vi "MISC Wait on Queue From Multiple.vi"(0 "Queue A":refnum<queue>, 5 "Queue B":refnum<queue>, 7 "timeout in ms (-1)":i32=-1, 11 "error in (no error)":errorcluster) -> (4 "Queue Element":string, 6 "Queue A?":bool, 8 "Queue B?":bool, 10 "Timed Out":bool, 15 "error Out":errorcluster)   [LabVIEW 2011]
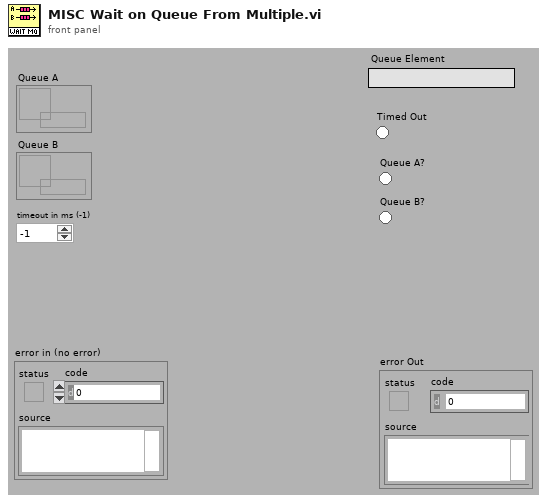
[diagram p1: front panel]
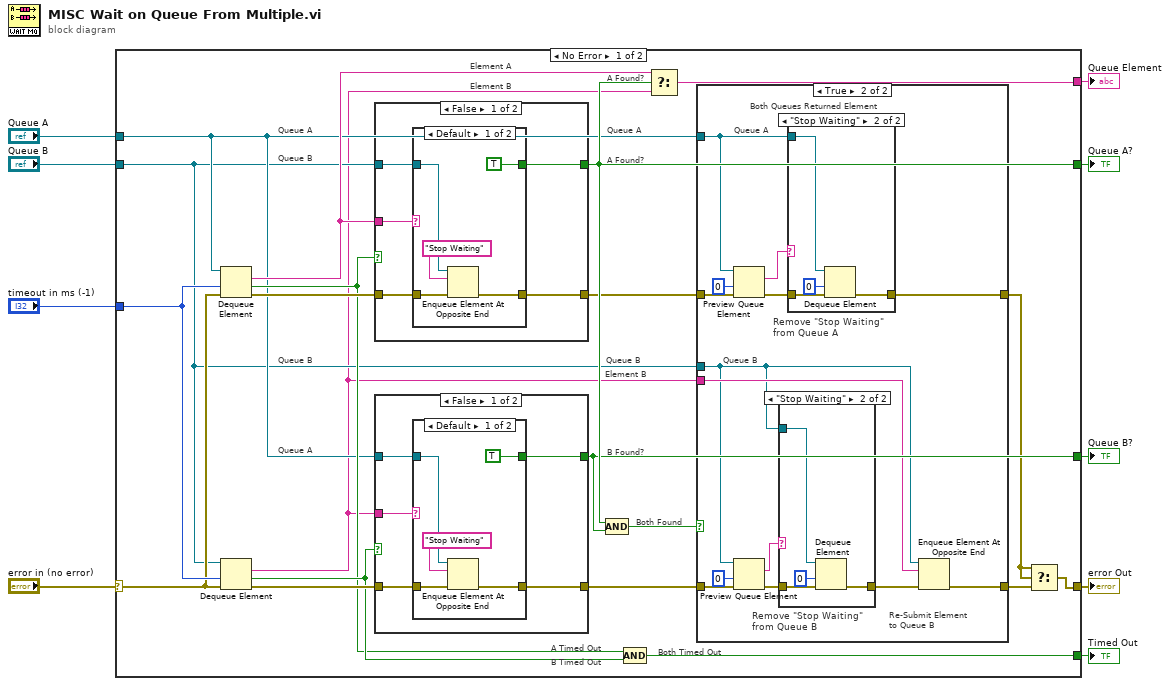
[diagram p0: block diagram]
diagram:
  n1 = case shown="No Error" "error in (no error)" {
    selector: "error in (no error)" -> [w28 w79]
    tunnel: "Queue B" -> [w14 _]
    tunnel: "Queue A" -> [w15 _]
    tunnel: "timeout in ms (-1)" -> [w29 _]
    tunnel: [w10 w79] -> w6
    tunnel: [w22 _] -> w4
    tunnel: [w21 _] -> w3
    tunnel: [w25 _] -> w2
    tunnel: [w23 _] -> w1
    frame No Error {
      # "Both Timed Out"
      # "Both Found"
      # "B Found?"
      # "Queue B"
      # "Element B"
      # "Queue A"
      # "A Found?"
      # "A Found?"
      # "Element B"
      # "Element A"
      # "B Timed Out"
      # "A Timed Out"
      # "Queue A"
      # "Queue B"
      # "Queue B"
      # "Queue A"
      n2 = Dequeue Element(queue=w15, timeout in ms (-1)=w29, error in (no error)=w28) -> (element=w24:string, timed out?=w18:bool, error out=w27:errorcluster)  [unwired: 1 out]
      n3 = Dequeue Element(queue=w14, timeout in ms (-1)=w29, error in (no error)=w28) -> (element=w13:string, timed out?=w19:bool, error out=w26:errorcluster)  [unwired: 1 out]
      n4 = case shown="False" w18 {
        tunnel: w14 -> [w71 _]
        tunnel: w27 -> [w70 w78]
        tunnel: w24 -> [w69 _]
        tunnel: [w68 w78] -> w17
        tunnel: [w67 _] -> w22
        frame False {
          n5 = case shown="Default" w69 {
            tunnel: w70 -> [w76 w77]
            tunnel: w71 -> [w75 _]
            tunnel: [w73 w77] -> w68
            tunnel: [TRUE _] -> w67
            frame Default {
              n6 = Enqueue Element At Opposite End(queue=w75, element="Stop Waiting", error in (no error)=w76) -> (error out=w73:errorcluster)  [unwired: 3 out]
            }
            frame "Stop Waiting" {
            }
          }
        }
        frame True {
        }
      }
      n7 = case shown="False" w19 {
        tunnel: w15 -> [w59 _]
        tunnel: w26 -> [w58 w66]
        tunnel: w13 -> [w57 _]
        tunnel: [w56 w66] -> w16
        tunnel: [w55 _] -> w21
        frame False {
          n8 = case shown="Default" w57 {
            tunnel: w58 -> [w64 w65]
            tunnel: w59 -> [w63 _]
            tunnel: [w61 w65] -> w56
            tunnel: [TRUE _] -> w55
            frame Default {
              n9 = Enqueue Element At Opposite End(queue=w63, element="Stop Waiting", error in (no error)=w64) -> (error out=w61:errorcluster)  [unwired: 3 out]
            }
            frame "Stop Waiting" {
            }
          }
        }
        frame True {
        }
      }
      n10 = Compound Arithmetic op=AND(w22, w21) -> (w20:bool)
      n11 = Compound Arithmetic op=AND(w18, w19) -> (w25:bool)
      n12 = Select(t=w24, s=w22, f=w13) -> (s? t:f=w23:string)
      n13 = case shown="True" w20 {
        tunnel: w16 -> [w31 w42]
        tunnel: [w31 w44] -> w11
        tunnel: w17 -> [w30 w43]
        tunnel: w15 -> [_ w38]
        tunnel: w14 -> [_ w33]
        tunnel: w13 -> [_ w41]
        tunnel: [w30 w37] -> w12
        frame False {
          # "0 or 1 Queues returned an Element"
        }
        frame True {
          # "Re-Submit Element to Queue B"
          # "Remove \"Stop Waiting\" from Queue A"
          # "Remove \"Stop Waiting\" from Queue B"
          # "Both Queues Returned Element"
          # "Queue B"
          # "Queue A"
          n14 = Preview Queue Element(queue=w38, timeout in ms (-1)=0, error in (no error)=w43) -> (element=w40:string, error out=w39:errorcluster)  [unwired: 2 out]
          n15 = Preview Queue Element(queue=w33, timeout in ms (-1)=0, error in (no error)=w42) -> (element=w32:string, error out=w34:errorcluster)  [unwired: 2 out]
          n16 = case shown="\"Stop Waiting\"" w32 {
            tunnel: w34 -> [w45 w49]
            tunnel: w33 -> [_ w48]
            tunnel: [w45 w46] -> _
            frame Default {
            }
            frame "Stop Waiting" {
              n17 = Dequeue Element(queue=w48, timeout in ms (-1)=0, error in (no error)=w49) -> (error out=w46:errorcluster)  [unwired: 3 out]
            }
          }
          n18 = case shown="\"Stop Waiting\"" w40 {
            tunnel: w39 -> [w50 w54]
            tunnel: w38 -> [_ w53]
            tunnel: [w50 w51] -> w37
            frame Default {
            }
            frame "Stop Waiting" {
              n19 = Dequeue Element(queue=w53, timeout in ms (-1)=0, error in (no error)=w54) -> (error out=w51:errorcluster)  [unwired: 3 out]
            }
          }
          n20 = Enqueue Element At Opposite End(queue=w33, element=w41, error in (no error)=w42) -> (error out=w44:errorcluster)  [unwired: 3 out]
        }
      }
      n21 = Select(t=w12, s=w12, f=w11) -> (s? t:f=w10:errorcluster)
    }
    frame Error {
    }
  }
  "Queue Element" <- w1
  "Timed Out" <- w2
  "Queue A?" <- w4
  "Queue B?" <- w3
  "error Out" <- w6
